vi "Main.vi"(11 "Module Admin":refnum<class "Delacor_lib_QMH_Module Admin.lvclass">) -> ()   [LabVIEW 2020, in "Acquisition.lvlib"]
doc: "This template is based off of the Queued Message Handler design pattern and the Queued Message Handler project template that ships with LabVIEW.\n\nThe main difference is that the queue is private to this module and communication between modules is performed via Broadcast and Request events.\n\nRequest events are wrapped in public API methods and are handled in the Event Handling Loop (EHL) of this VI. Any module can register for Broadcast events sent by this module. The EHL generates messages based on user interface actions.\n\nThe Message Handling Loop (MHL) processes messages generated by the EHL, or by other messages. The messages are string values, so new messages can be added easily to the Message Cases case structure in the MHL. Each message cluster can also provide an optional value for Message Data, which is a variant that can be converted to whatever message-specific data is required.\n_____\nBased on Delacor QMH Project Template 5.0.0.82."
uses:
  Acquisition.lvlib
  <vilib>/Delacor/Delacor QMH/Libraries/Module Admin_class/Delacor_lib_QMH_Module Admin.lvclass
  Module Data--cluster.ctl
  SignalConfig--cluster.ctl
  Stop Argument--cluster.ctl
  <vilib>/Delacor/Delacor QMH/Libraries/Message Queue_class/Delacor_lib_QMH_Message Queue.lvclass/Delacor_lib_QMH_Message Queue.ctl
  <vilib>/Delacor/Delacor QMH/Libraries/Module Admin_class/Delacor_lib_QMH_Module Admin.lvclass/Delacor_lib_QMH_Module Admin.ctl
  Start AQ Argument--cluster.ctl
  Stop AQ Argument--cluster.ctl
  Set AQ parameters Argument--cluster.ctl
  <vilib>/Utility/miscctls.llb/LVPointTypeDef.ctl
  <vilib>/Delacor/Delacor QMH/Libraries/Message Queue_class/Delacor_lib_QMH_Enqueue Message (Single).vi
  <vilib>/Delacor/Delacor QMH/Libraries/Module Admin_class/Delacor_lib_QMH_Get External Launch.vi
  <vilib>/Utility/error.llb/Error Cluster From Error Code.vi
  <vilib>/ErrorRing/Error Ring.xnode
  <vilib>/Delacor/Delacor QMH/Libraries/Message Queue_class/Delacor_lib_QMH_Message Queue.lvclass
  <vilib>/measure/NI_MABase.lvlib
  <vilib>/Analysis/NI_AALBase.lvlib
panel:
  out "error out":errorcluster
  out "Status":string
types:
  T1 = typedef "Acquisition.lvlib/Request Events--cluster.ctl" = cluster{"Stop Module":refnum<user-event>, "Show Panel":refnum<user-event>, "Hide Panel":refnum<user-event>, "Get Module Execution Status":refnum<user-event>, "Show Diagram":refnum<user-event>, "Start AQ":refnum<user-event>, "Stop AQ":refnum<user-event>, "Wake Up HL":refnum<user-event>, "Put HL to Sleep":refnum<user-event>, "Set AQ parameters":refnum<user-event>}
  T2 = typedef "Acquisition.lvlib/Module Data--cluster.ctl" = cluster{"Status":string, "TimeOut":i32, "SignalConfig":T3}
  T3 = typedef "SignalConfig--cluster.ctl" = cluster{"VPP":i32, "Frecuency":dbl, "Offset":dbl, "signal type":enum16{"Sine Wave", "Triangle Wave", "Square Wave", "Sawtooth Wave"}}
  T4 = enum32{"invalid lock state", "Not Locked", "Locked (No Password)", "Password-protected"}
  T5 = typedef "Acquisition.lvlib/Stop Argument--cluster.ctl" = cluster{"Origin":string, "Exit via Stop Module Req?":bool, "Wait for Module to stop?":bool}
  T6 = typedef "Acquisition.lvlib/Start AQ Argument--cluster.ctl" = cluster{"Boolean":bool}
  T7 = typedef "Acquisition.lvlib/Stop AQ Argument--cluster.ctl" = cluster{"Boolean":bool}
  T8 = typedef "Acquisition.lvlib/Set AQ parameters Argument--cluster.ctl" = cluster{"SignalConfig":T3}
  T9 = typedef "LVPointTypeDef.ctl" = cluster{"Horizontal":i16, "Vertical":i16}
  T10 = enum32{"Invalid", "Standard", "Closed", "Hidden", "Minimized", "Maximized"}
  T11 = enum16{"Sine Wave", "Triangle Wave", "Square Wave", "Sawtooth Wave"}
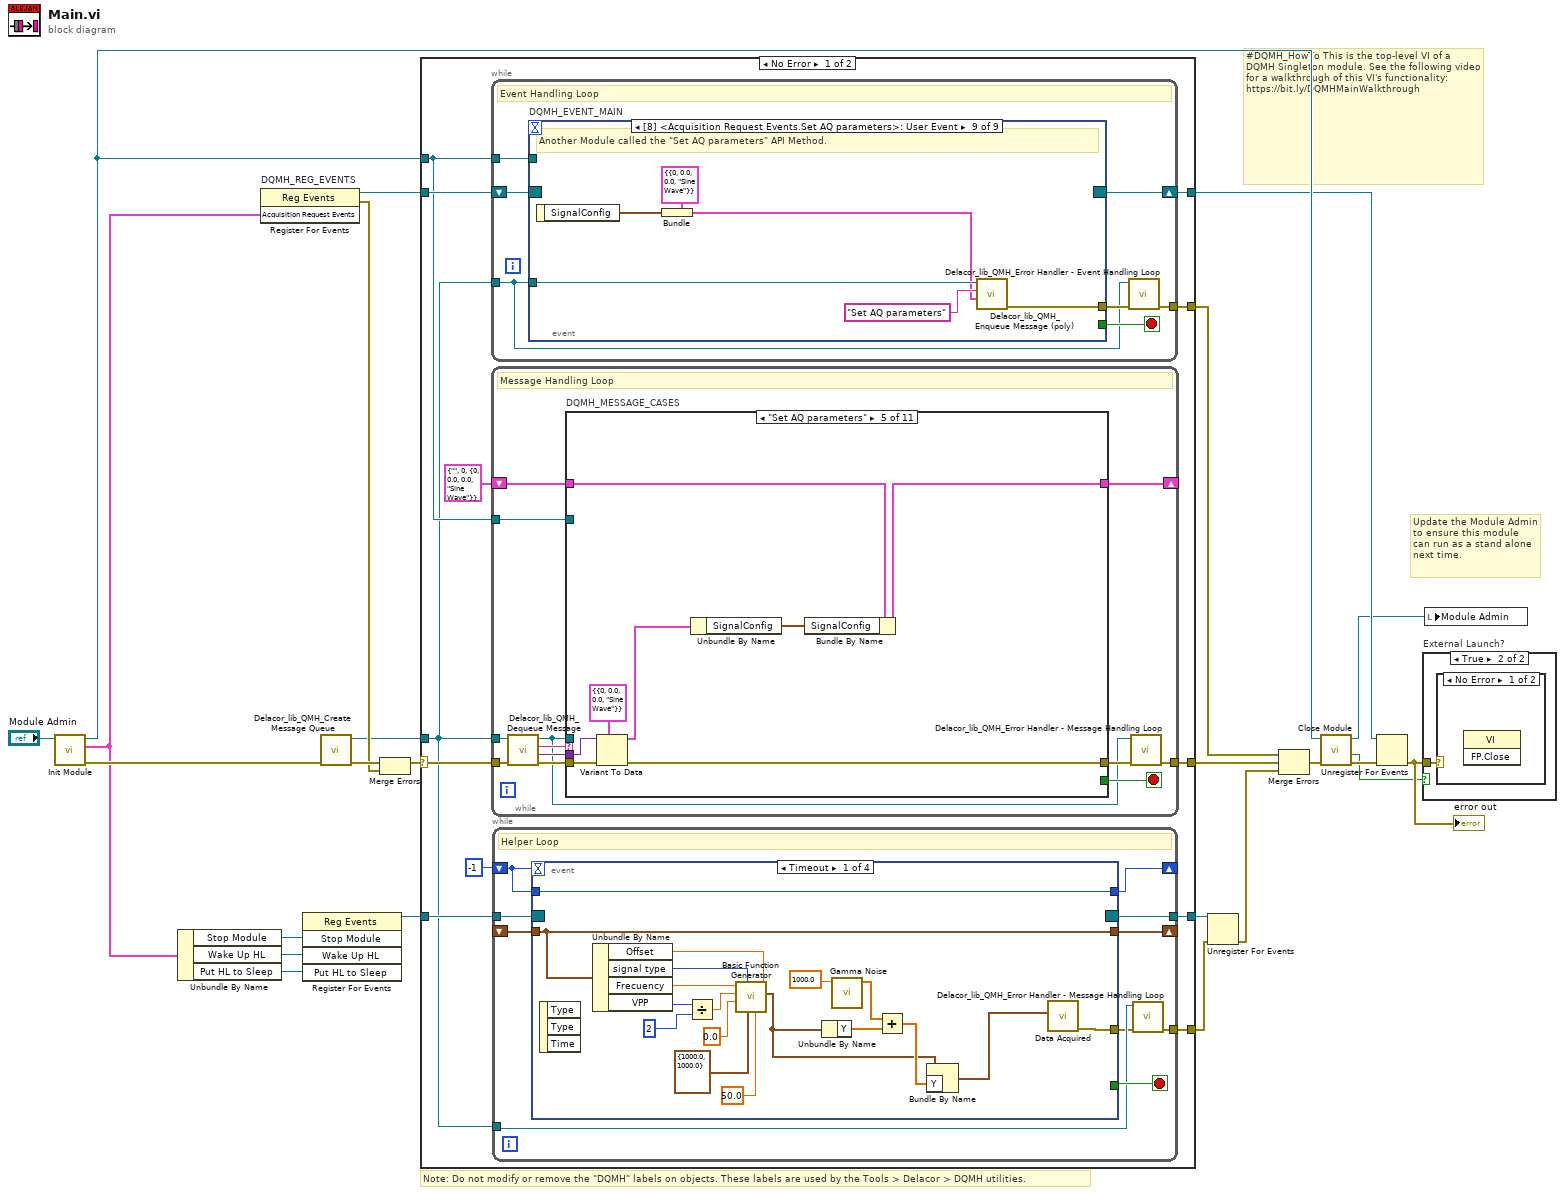
[diagram p0: block diagram]
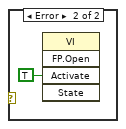
[diagram p3: hidden frame]
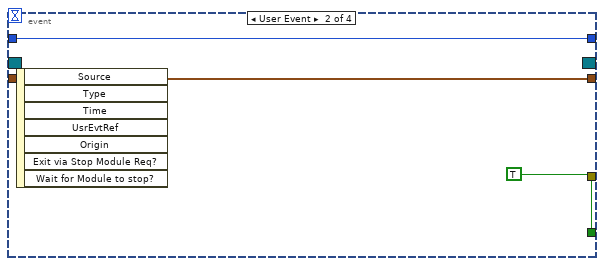
[diagram p4: hidden frame]
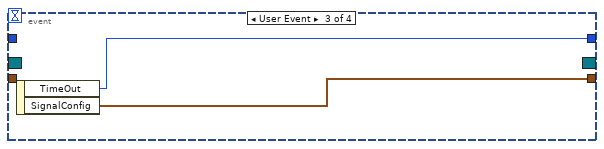
[diagram p5: hidden frame]
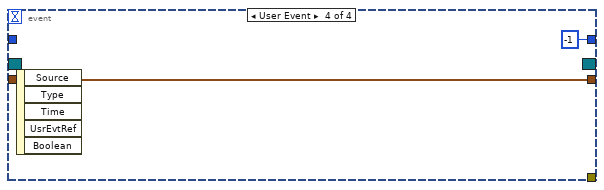
[diagram p6: hidden frame]
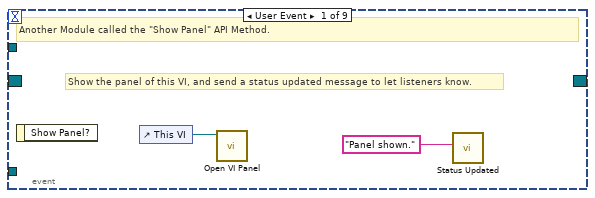
[diagram p7: hidden frame]
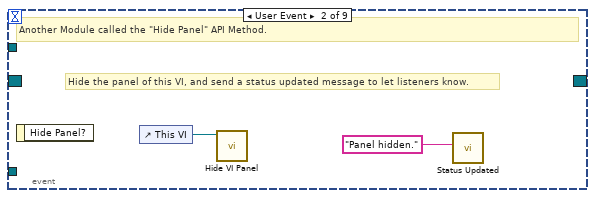
[diagram p8: hidden frame]
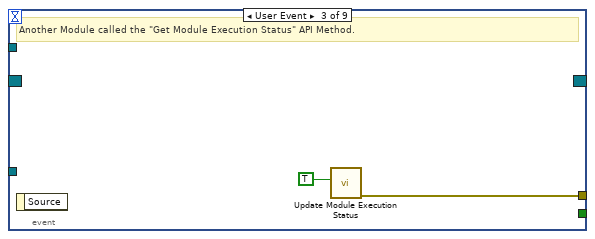
[diagram p9: hidden frame]
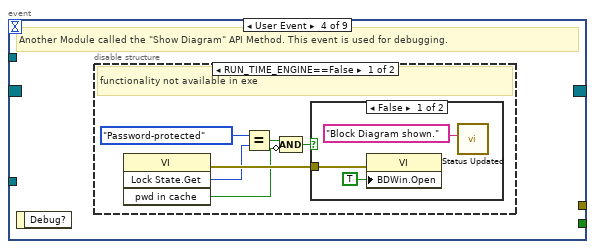
[diagram p10: hidden frame]
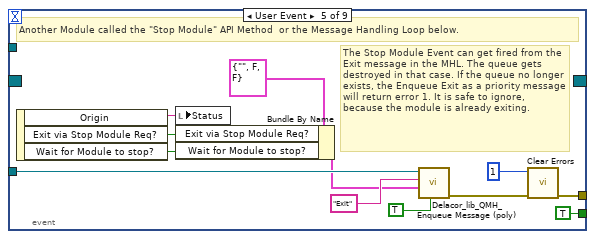
[diagram p13: hidden frame]
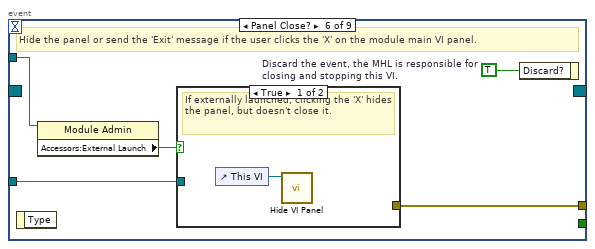
[diagram p14: hidden frame]
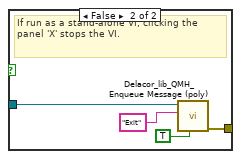
[diagram p15: hidden frame]
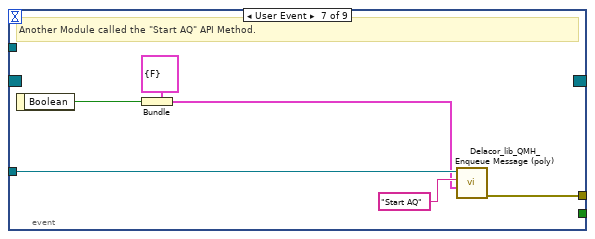
[diagram p16: hidden frame]
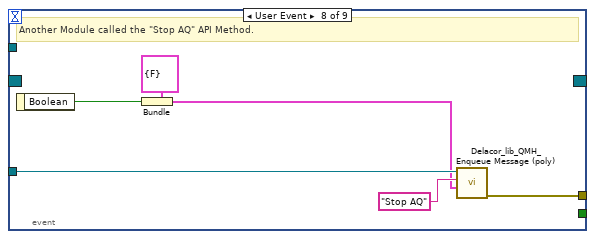
[diagram p17: hidden frame]
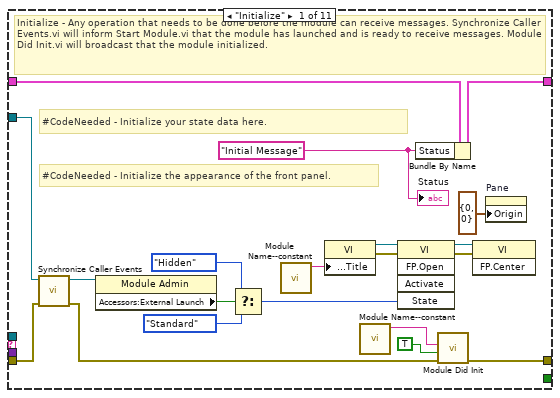
[diagram p18: hidden frame]
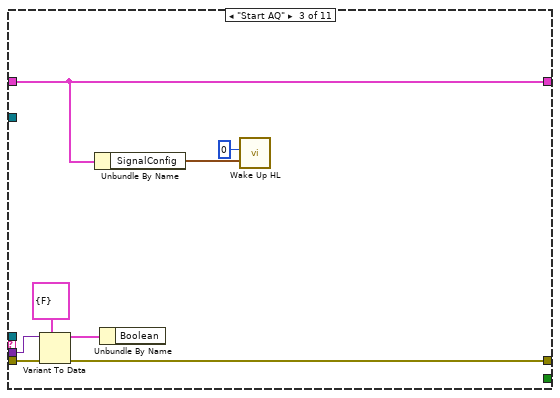
[diagram p20: hidden frame]
diagram:
  # "#DQMH_HowTo This is the top-level VI of a DQMH Singleton module. See the following video for a walkthrough of this VI's functionality: https://bit.ly/DQMHMainWalkthrough"
  # "Note: Do not modify or remove the \"DQMH\" labels on objects. These labels are used by the Tools > Delacor > DQMH utilities."
  # "Update the Module Admin to ensure this module can run as a stand alone next time."
  n1 = call "Init Module.vi"("Singleton Module Admin in"="Module Admin") -> ("error out"=w23:errorcluster, "Acquisition Request Events"=w4:T1, "Singleton Module Admin out"=w15:refnum<class "Delacor_lib_QMH_Module Admin.lvclass">)  [unwired: 8 in]
  n2 = Unbundle By Name(w4) -> ("Stop Module"=w3:refnum<user-event>, "Wake Up HL"=w2:refnum<user-event>, "Put HL to Sleep"=w1:refnum<user-event>)
  n3 = register-events "DQMH_REG_EVENTS"(w4) -> (reference out=w13:refnum<event-registration>, error out=w16:errorcluster)  [unwired: 2 in]
  n4 = register-events(w3, w2, w1) -> (reference out=w5:refnum<event-registration>)  [unwired: 2 in, 1 out]
  n5 = call <vilib>:"Delacor_lib_QMH_Create Message Queue.vi"("error in"=w23) -> ("error out"=w18:errorcluster, "Message Queue"=w12:refnum<class "Delacor_lib_QMH_Message Queue.lvclass">)  [unwired: 9 in]
  n6 = Merge Errors(w18, w16) -> (w17:errorcluster)
  n7 = case shown="No Error" w17 {
    selector: w17 -> [w34 w252]
    tunnel: [w36 w251] -> w24
    tunnel: [w33 w257] -> w14
    tunnel: w13 -> [w31 w257]
    tunnel: w12 -> [w25 w250]
    tunnel: [w35 _] -> w21
    tunnel: w15 -> [w30 w253]
    tunnel: [w28 _] -> w6
    tunnel: [w27 w249] -> w8
    tunnel: w5 -> [w26 w249]
    frame No Error {
      n8 = while {
        tunnel: w25 -> [w72]
        shift-right: [w75] -> w33
        shift-left: w31 -> [w76]
        tunnel: [w77] -> w35
        tunnel: w30 -> [w73]
        stop <- w74 stop-if-true
        # "Event Handling Loop"
        n9 = event "DQMH_EVENT_MAIN" shown="[8] <Acquisition Request Events.Set AQ parameters>: User Event" {
          selector: w76 -> [_ _ _ _ _ _ _ _ _]
          dyn-events: [_ _ _ _ _ _ _ _ _] -> w75
          timeout: _ -> [_ _ _ _ _ _ _ _ _]
          tunnel: [_ _ _ _ TRUE ("Discard?") _ _ _ _] -> w74
          tunnel: w72 -> [_ _ _ _ w101 w108 w121 w127 w133]
          tunnel: [_ _ w84 _ w104 w110 w116 w122 w128] -> w78
          tunnel: w73 -> [_ _ _ _ _ w107 _ _ _]
          event User Event {
            # "Show the panel of this VI, and send a status updated message to let listeners know."
            # "Another Module called the \"Show Panel\" API Method."
            n10 = event-data() -> ()  [unwired: 1 in, 1 out]
            n11 = control-ref of="This VI"() -> (w80:refnum<vi>)
            n12 = call "Open VI Panel.vi"("VI"=w80) -> ()  [unwired: 10 in, 1 out]
            n13 = call "Status Updated.vi"("Status"="Panel shown." ("format string")) -> ()  [unwired: 10 in, 1 out]
          }
          event User Event {
            # "Hide the panel of this VI, and send a status updated message to let listeners know."
            # "Another Module called the \"Hide Panel\" API Method."
            n14 = event-data() -> ()  [unwired: 1 in, 1 out]
            n15 = control-ref of="This VI"() -> (w82:refnum<vi>)
            n16 = call "Hide VI Panel.vi"("VI"=w82) -> ()  [unwired: 10 in, 1 out]
            n17 = call "Status Updated.vi"("Status"="Panel hidden." ("format string")) -> ()  [unwired: 10 in, 1 out]
          }
          event User Event {
            # "Another Module called the \"Get Module Execution Status\" API Method."
            n18 = event-data() -> ()  [unwired: 1 in, 1 out]
            n19 = call "Update Module Execution Status.vi"("Running?"=TRUE) -> ("error out"=w84:errorcluster)  [unwired: 10 in]
          }
          event User Event {
            # "Another Module called the \"Show Diagram\" API Method. This event is used for debugging."
            n20 = event-data() -> ()  [unwired: 1 in, 1 out]
            n21 = disable-structure shown="RUN_TIME_ENGINE==False" {
              frame condition #0 (active) {
                # "functionality not available in exe"
                n22 = invoke class="VI" method="Lock State.Get"() -> (error out=w90:errorcluster, "Get Lock State"=w89:T4, "pwd in cache"=w86:bool)  [unwired: 4 in, 1 out]
                n23 = Equal?(x=T4."Password-protected", y=w89) -> (x = y?=w87:bool)
                n24 = Compound Arithmetic op=AND(w87, invert w86) -> (w85:bool)
                n25 = case shown="False" w85 {
                  tunnel: w90 -> [w93 _]
                  frame False {
                    n26 = property class="VI"(error in=w93, "BDWin.Open"=TRUE ("Block Diagram Window:Open")) -> ()  [unwired: 1 in, 2 out]
                    n27 = call "Status Updated.vi"("Status"="Block Diagram shown." ("format string")) -> ()  [unwired: 10 in, 1 out]
                  }
                  frame True {
                    # "Password-protected VI, and the password is not in the cache. Do not show the diagram."
                  }
                }
              }
              frame condition #1 {
              }
            }
          }
          event User Event {
            # "The Stop Module Event can get fired from the Exit message in the MHL. The queue gets destroyed in that case. If the queue no longer exists, the Enqueue Exit as a priority message will return error 1. It is safe to ignore, because the module is already exiting."
            # "Another Module called the \"Stop Module\" API Method  or the Message Handling Loop below."
            n28 = event-data() -> ("Origin"=w100:string, "Exit via Stop Module Req?"=w96:bool, "Wait for Module to stop?"=w95:bool)  [unwired: 1 in]
            n29 = local write "Status"(w100) -> ()
            n30 = Bundle By Name(cluster=T5 {"Origin"="", "Exit via Stop Module Req?"=FALSE, "Wait for Module to stop?"=FALSE} ("Stop Argument"), "Exit via Stop Module Req?"=w96, "Wait for Module to stop?"=w95) -> (w94:T5)
            n31 = call-poly <vilib>:"Delacor_lib_QMH_Enqueue Message (poly).vi"("Priority Message? (F)"=TRUE, "Message Data"=w94, "Message"="Exit", "Message Queue in"=w101) -> ("error out"=w105:errorcluster)  [unwired: 6 in, 1 out]
            n32 = call <vilib>:"Clear Errors.vi"("error in (no error)"=w105, "specific error code to clear (0: all)"=1) -> ("error out"=w104:errorcluster)  [unwired: 4 in, 1 out]
          }
          event Panel Close? {
            w109 = TRUE  # Discard the event, the MHL is responsible for closing and stopping this VI.
            # "Hide the panel or send the 'Exit' message if the user clicks the 'X' on the module main VI panel."
            n33 = event-data() -> ()  [unwired: 1 in, 1 out]
            n34 = property class="Module Admin"(reference=w107) -> ("Accessors:External Launch"=w106:bool)  [unwired: 1 in, 2 out]
            n35 = case shown="True" w106 {
              tunnel: w108 -> [_ w114]
              tunnel: [_ w115] -> w110
              frame True {
                # "If externally launched, clicking the 'X' hides the panel, but doesn't close it."
                n36 = control-ref of="This VI"() -> (w111:refnum<vi>)
                n37 = call "Hide VI Panel.vi"("VI"=w111) -> ()  [unwired: 10 in, 1 out]
              }
              frame False {
                # "If run as a stand-alone VI, clicking the panel 'X' stops the VI."
                n38 = call-poly <vilib>:"Delacor_lib_QMH_Enqueue Message (poly).vi"("Priority Message? (F)"=TRUE, "Message"="Exit", "Message Queue in"=w114) -> ("error out"=w115:errorcluster)  [unwired: 7 in, 1 out]
              }
            }
            n39 = event-data("Discard?"=w109) -> ()  [unwired: 1 in, 1 out]
          }
          event User Event {
            # "Another Module called the \"Start AQ\" API Method."
            n40 = event-data() -> ("Boolean"=w117:bool)  [unwired: 1 in]
            n41 = Bundle(cluster=T6 {"Boolean"=FALSE} ("Start AQ Argument"), "Boolean"=w117) -> (w118:T6)
            n42 = call-poly <vilib>:"Delacor_lib_QMH_Enqueue Message (poly).vi"("Message Data"=w118, "Message"="Start AQ", "Message Queue in"=w121) -> ("error out"=w116:errorcluster)  [unwired: 7 in, 1 out]
          }
          event User Event {
            # "Another Module called the \"Stop AQ\" API Method."
            n43 = event-data() -> ("Boolean"=w123:bool)  [unwired: 1 in]
            n44 = Bundle(cluster=T7 {"Boolean"=FALSE} ("Stop AQ Argument"), "Boolean"=w123) -> (w124:T7)
            n45 = call-poly <vilib>:"Delacor_lib_QMH_Enqueue Message (poly).vi"("Message Data"=w124, "Message"="Stop AQ", "Message Queue in"=w127) -> ("error out"=w122:errorcluster)  [unwired: 7 in, 1 out]
          }
          event User Event {
            # "Another Module called the \"Set AQ parameters\" API Method."
            n46 = event-data() -> ("SignalConfig"=w129:T3)  [unwired: 1 in]
            n47 = Bundle(cluster=T8 {"SignalConfig"={"VPP"=0, "Frecuency"=0.0, "Offset"=0.0, "signal type"=enum."Sine Wave"}} ("Set AQ parameters Argument"), "SignalConfig"=w129) -> (w130:T8)
            n48 = call-poly <vilib>:"Delacor_lib_QMH_Enqueue Message (poly).vi"("Message Data"=w130, "Message"="Set AQ parameters", "Message Queue in"=w133) -> ("error out"=w128:errorcluster)  [unwired: 7 in, 1 out]
          }
        }
        n49 = call-dynamic "Delacor_lib_QMH_Error Handler - Event Handling Loop.vi"("error in"=w78, "Message Queue in"=w72) -> ("dup error in"=w77:errorcluster)  [unwired: 8 in, 1 out]
      }
      n50 = while {
        tunnel: w25 -> [w136]
        shift-right: [w140] -> _
        shift-left: T2 {"Status"="", "TimeOut"=0, "SignalConfig"={"VPP"=0, "Frecuency"=0.0, "Offset"=0.0, "signal type"=enum."Sine Wave"}} ("Data Cluster") -> [w141]
        tunnel: w34 -> [w144]
        tunnel: [w142] -> w36
        tunnel: w30 -> [w134]
        stop <- w139 stop-if-true
        # "Message Handling Loop"
        n51 = call-dynamic "Delacor_lib_QMH_Dequeue Message.vi"("error in"=w144, "Message Queue in"=w136) -> ("error out"=w143:errorcluster, "Message Data"=w137:variant, "Message"=w138:string, "Message Queue out"=w135:refnum<class "Delacor_lib_QMH_Message Queue.lvclass">)  [unwired: 6 in]
        n52 = case "DQMH_MESSAGE_CASES" shown="\"Set AQ parameters\"" w138 {
          selector: w138 -> [_ _ _ _ _ _ _ _ _ _ w236]
          tunnel: w135 -> [_ _ _ _ _ _ _ _ w206 w228 _]
          tunnel: w143 -> [w163 w167 w175 w176 w186 w189 w191 w196 w213 w234 w238]
          tunnel: [w161 w167 w174 w177 w184 w188 w191 w195 w209 w231 w239] -> w145
          tunnel: w141 -> [w152 w166 w170 w178 w185 w187 w190 w193 w208 w227 w237]
          tunnel: [w151 w166 w170 w178 w180 w187 w190 w193 w208 w227 w237] -> w140
          tunnel: [_ _ _ _ _ _ _ _ _ w226 _] -> w139
          tunnel: w137 -> [_ _ w173 _ w183 _ _ _ w207 w225 _]
          tunnel: w134 -> [w153 _ _ _ _ _ _ _ w205 w220 _]
          frame "Initialize" {
            w146 = "Initial Message" ("Initial Message")
            # "#CodeNeeded - Initialize the appearance of the front panel."
            # "#CodeNeeded - Initialize your state data here."
            # "Initialize - Any operation that needs to be done before the module can receive messages. Synchronize Caller Events.vi will inform Start Module.vi that the module has launched and is ready to receive messages. Module Did Init.vi will broadcast that the module initialized."
            n53 = call "Synchronize Caller Events.vi"("error in (no error)"=w163, "Singleton Module Admin in"=w153) -> ("error out"=w162:errorcluster, "Singleton Module Admin out"=w148:refnum<class "Delacor_lib_QMH_Module Admin.lvclass">)  [unwired: 8 in]
            n54 = property class="Module Admin"(reference=w148) -> ("Accessors:External Launch"=w157:bool)  [unwired: 1 in, 2 out]
            n55 = Select(t=T10."Hidden" ("State"), s=w157, f=T10."Standard" ("State")) -> (s? t:f=w154:T10)
            n56 = call "Module Name--constant.vi"() -> ("Module Name"=w160:string)  [unwired: 11 in]
            n57 = property class="VI"("Front Panel.Title"=w160) -> (reference out=w159:refnum<vi>, error out=w165:errorcluster)  [unwired: 2 in]
            n58 = call "Module Name--constant.vi"() -> ("Module Name"=w149:string)  [unwired: 11 in]
            n59 = invoke class="VI" method="FP.Open"(reference=w159, error in=w165, "State"=w154) -> (reference out=w158:refnum<vi>, error out=w164:errorcluster)  [unwired: 2 in, 3 out]
            n60 = Bundle By Name(cluster=w152, "Status"=w146) -> (w151:T2)
            n61 = call "Module Did Init.vi"("error in (no error)"=w162, "Initialized?"=TRUE, "Origin"=w149) -> ("error out"=w161:errorcluster)  [unwired: 8 in]
            n62 = invoke class="VI" method="FP.Center"(reference=w158, error in=w164) -> ()  [unwired: 1 in, 3 out]
            n63 = property on="Pane" class="Pane"("Origin"=T9 {"Horizontal"=0, "Vertical"=0}) -> ()  [unwired: 2 in, 2 out]
            "Status" <- w146
          }
          frame "--- Module Specific ---" {
            # "Separator -- The following cases handle messages specific to this Module."
          }
          frame "Start AQ" {
            n64 = Variant To Data(error in=w175, type=T6 {"Boolean"=FALSE} ("Start AQ Argument"), Variant=w173) -> (data=w171:T6, error out=w174:errorcluster)
            n65 = Unbundle By Name(w170) -> ("SignalConfig"=w169:T3)
            n66 = Unbundle By Name(w171) -> ()  [unwired: 1 out]
            n67 = call "Wake Up HL.vi"("SignalConfig"=w169, "TimeOut"=0) -> ()  [unwired: 9 in, 1 out]
          }
          frame "Stop AQ" {
            n68 = call "Put HL to Sleep.vi"("error in"=w176) -> ("error out"=w177:errorcluster)  [unwired: 10 in]
          }
          frame "Set AQ parameters" {
            n69 = Variant To Data(error in=w186, type=T8 {"SignalConfig"={"VPP"=0, "Frecuency"=0.0, "Offset"=0.0, "signal type"=enum."Sine Wave"}} ("Set AQ parameters Argument"), Variant=w183) -> (data=w181:T8, error out=w184:errorcluster)
            n70 = Unbundle By Name(w181) -> ("SignalConfig"=w179:T3)
            n71 = Bundle By Name(cluster=w185, "SignalConfig"=w179) -> (w180:T2)
          }
          frame "---Copy This Frame---" {
            # "Duplicate this frame when creating new messages.  Change this comment in the duplicated frame to describe this message."
            n72 = Merge Errors(w189) -> (w188:errorcluster)
          }
          frame "--- Exit and Error Handling---" {
            # "Separator - The following cases handle errors and exit messages."
          }
          frame "Simulate MHL Error" {
            # "#DQMH_HowTo The 'Simulate MHL Error' button  illustrates how the MHL handles errors. This event is instructional in nature and can be removed."
            # "Simulate an error occurring at the MHL"
            n73 = call "Module Name--constant.vi"() -> ("Module Name"=w192:string)  [unwired: 11 in]
            n74 = xnode "Error Ring"("parameter 0"=w192) -> ("error out"=w194:errorcluster)
            n75 = Merge Errors(w196, w194) -> (w195:errorcluster)
          }
          frame "Error" {
            # "#CodeRecommended - If you ever change the name of this \"Error\" message, you'll need to update the name in the Check Loop Error.vi as well."
            # "#CodeRecommended - If the module is running in standalone mode (External Launch = FALSE), this code will pop up an error dialog and call the 'Exit' message if an error occurs. Add more fine-grained error handling here."
            # "Error - Check the error message data and respond accordingly. This message is sent by the \"Error Handler\" VIs at the end of each loop in this application."
            n76 = property class="Module Admin"(reference=w205) -> ("Accessors:External Launch"=w204:bool)  [unwired: 1 in, 2 out]
            n77 = Variant To Data(error in=w213, type=errorcluster {"status"=FALSE, "code"=0, "source"=""} ("error constant"), Variant=w207) -> (data=w214:errorcluster, error out=w211:errorcluster)
            n78 = call "Error Reported.vi"("Error"=w214) -> ()  [unwired: 10 in, 1 out]
            n79 = case shown="False" w204 {
              tunnel: [w219 _] -> w210
              tunnel: w206 -> [w217 _]
              tunnel: w214 -> [w218 _]
              frame False {
                # "If the module is running standalone, then pop up an error dialog and call the \"Exit\" message."
                n80 = call <vilib>:"Simple Error Handler.vi"("error in (no error)"=w218) -> ()  [unwired: 4 in, 5 out]
                n81 = call-poly <vilib>:"Delacor_lib_QMH_Enqueue Message (poly).vi"("Priority Message? (F)"=TRUE, "Message"="Exit", "Message Queue in"=w217) -> ("error out"=w219:errorcluster)  [unwired: 7 in, 1 out]
              }
              frame True {
                # "If the module was launched externally, calling the Error Reported broadcast VI is the only action performed by the \"Error\" message. The module's caller can then process the error appropriately."
              }
            }
            n82 = Merge Errors(w211, w210) -> (w209:errorcluster)
            n83 = local write "error out"(w209) -> ()
          }
          frame "Exit" {
            w224 = 91  # 91: not all Exit messages will have an argument
            w226 = TRUE  # Stop the VI
            # "Release the message queue reference"
            # "#CodeNeeded - Add any required cleanup code here"
            # "Exit - Exit the application."
            n84 = Variant To Data(error in=w234, type=T5 {"Origin"="", "Exit via Stop Module Req?"=FALSE, "Wait for Module to stop?"=FALSE} ("Stop Argument"), Variant=w225) -> (data=w222:T5, error out=w230:errorcluster)
            n85 = call <vilib>:"Clear Errors.vi"("error in (no error)"=w230, "specific error code to clear (0: all)"=w224) -> ("error out"=w233:errorcluster)  [unwired: 4 in, 1 out]
            n86 = control-ref of="This VI"() -> (w221:refnum<vi>)
            n87 = call-dynamic "Delacor_lib_QMH_Release Message Queue.vi"("error in"=w233, "Message Queue"=w228) -> ("error out"=w232:errorcluster)  [unwired: 9 in]
            n88 = call "Handle Exit.vi"("Stop Argument"=w222, "Admin in"=w220, "VI reference"=w221) -> ("error out"=w229:errorcluster)  [unwired: 7 in, 1 out]
            n89 = Merge Errors(w232, w229) -> (w231:errorcluster)
          }
          frame Default {
            # "'Default' case only runs if there is a message that isn't defined in any of the other cases.  Output a programming error."
            n90 = call "Module Name--constant.vi"() -> ("Module Name"=w235:string)  [unwired: 11 in]
            n91 = xnode "Error Ring"("parameter 0"=w236, "parameter 1"=w235) -> ("error out"=w240:errorcluster)
            n92 = Merge Errors(w238, w240) -> (w239:errorcluster)
          }
        }
        n93 = call-dynamic "Delacor_lib_QMH_Error Handler - Message Handling Loop.vi"("error in"=w145, "Message Queue in"=w135) -> ("dup error in"=w142:errorcluster)  [unwired: 8 in, 1 out]
      }
      n94 = while {
        shift-right: [w45] -> _
        shift-left: -1 -> [w46]
        tunnel: [w44] -> w28
        tunnel: [w43] -> w27
        tunnel: w26 -> [w42]
        tunnel: w25 -> [w40]
        shift-right: [w39] -> _
        shift-left: _ -> [w38]
        stop <- w41 stop-if-true
        # "Helper Loop"
        n95 = event shown="[0] Timeout" {
          selector: w42 -> [_ _ _ _]
          dyn-events: [_ _ _ _] -> w43
          timeout: w46 -> [_ _ _ _]
          tunnel: [w64 w65 w69 -1 ("TimeOut")] -> w45
          tunnel: w46 -> [w64 w65 _ _]
          tunnel: [_ TRUE _ _] -> w41
          tunnel: [w63 w66 w68 w71] -> w39
          tunnel: w38 -> [w63 w66 _ w71]
          tunnel: [w56 _ _ _] -> w37
          event Timeout {
            n96 = event-data() -> ()  [unwired: 1 in, 3 out]
            n97 = Unbundle By Name(w63) -> ("Offset"=w61:dbl, "signal type"=w62:T11, "Frecuency"=w60:dbl, "VPP"=w59:i32)
            n98 = Divide(x=w59, y=2) -> (x/y=w58:dbl)
            n99 = call <vilib>:"Basic Function Generator.vi"("offset"=w61, "square wave duty cycle (%)"=50.0, "sampling info"=cluster{"Fs":dbl, "#s":dbl} {"Fs"=1000.0, "#s"=1000.0}, "signal type"=w62, "phase"=0.0, "amplitude"=w58, "frequency"=w60) -> ("signal out"=w48:waveform(dbl))  [unwired: 2 in, 2 out]
            n100 = Unbundle By Name(w48) -> ("Y"=w50:dbl[])
            n101 = call <vilib>:"Gamma Noise.vi"("samples"=1000.0) -> ("gamma noise"=w49:dbl[])  [unwired: 9 in, 1 out]
            n102 = Add(x=w49, y=w50) -> (x+y=w52:dbl[])
            n103 = Bundle By Name(cluster=w48, "Y"=w52) -> (w47:waveform(dbl))
            n104 = call "Data Acquired.vi"("DataAcquired"=w47) -> ("error out"=w56:errorcluster)  [unwired: 10 in]
          }
          event User Event {
            n105 = event-data() -> ()  [unwired: 1 in, 7 out]
          }
          event User Event {
            n106 = event-data() -> ("TimeOut"=w69:i32, "SignalConfig"=w68:T3)  [unwired: 1 in]
          }
          event User Event {
            n107 = event-data() -> ()  [unwired: 1 in, 5 out]
          }
        }
        n108 = call-dynamic "Delacor_lib_QMH_Error Handler - Message Handling Loop.vi"("error in"=w37, "Message Queue in"=w40) -> ("dup error in"=w44:errorcluster)  [unwired: 8 in, 1 out]
      }
    }
    frame Error {
      # "Synchronize Caller Events.vi will inform Start Module.vi that the module has launched and will let the code calling Start Module.vi register for broadcasts and would permit the caller receive the broadcast that an error occurred at launch time."
      n109 = call-dynamic "Delacor_lib_QMH_Release Message Queue.vi"("error in"=w252, "Message Queue"=w250) -> ("error out"=w251:errorcluster)  [unwired: 9 in]
      n110 = call "Synchronize Caller Events.vi"("Singleton Module Admin in"=w253) -> ("error out"=w258:errorcluster)  [unwired: 9 in, 1 out]
      n111 = call "Module Name--constant.vi"() -> ("Module Name"=w256:string)  [unwired: 11 in]
      n112 = Format Into String(format string="An error occurred during initialization. %s is no longer running.", w256) -> (resulting string=w254:string)  [unwired: 2 in, 1 out]
      n113 = Merge Errors(w251, w258) -> (w259:errorcluster)
      n114 = call "Error Reported.vi"("Additional Information"=w254, "Error"=w259) -> ()  [unwired: 9 in, 1 out]
    }
  }
  n115 = Unregister For Events(event registration refnum=w8, error in=w6) -> (error out=w7:errorcluster)
  n116 = Merge Errors(w21, w24, w7) -> (w20:errorcluster)
  n117 = call "Close Module.vi"("error in (no error)"=w20, "Module Admin in"=w15) -> ("error out"=w22:errorcluster, "External Launch"=w9:bool, "Module Admin out"=w10:refnum<class "Delacor_lib_QMH_Module Admin.lvclass">)  [unwired: 7 in]
  n118 = Unregister For Events(event registration refnum=w14, error in=w22) -> (error out=w19:errorcluster)
  "error out" <- w19
  n119 = case "External Launch?" shown="True" w9 {
    tunnel: w19 -> [_ w260]
    frame False {
    }
    frame True {
      n120 = case shown="No Error" w260 {
        frame No Error {
          n121 = invoke class="VI" method="FP.Close"() -> ()  [unwired: 3 in, 3 out]
        }
        frame Error {
          n122 = invoke class="VI" method="FP.Open"("Activate"=TRUE ("Activate?")) -> ()  [unwired: 4 in, 5 out]
        }
      }
    }
  }
  n123 = local write "Module Admin"(w10) -> ()
